vi "create_base_path.vi"(8 "folder name":string, 11 "folder":path) -> (3 "appended path":path)   [LabVIEW 2021]
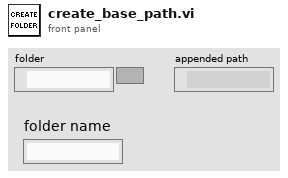
[diagram p1: front panel]
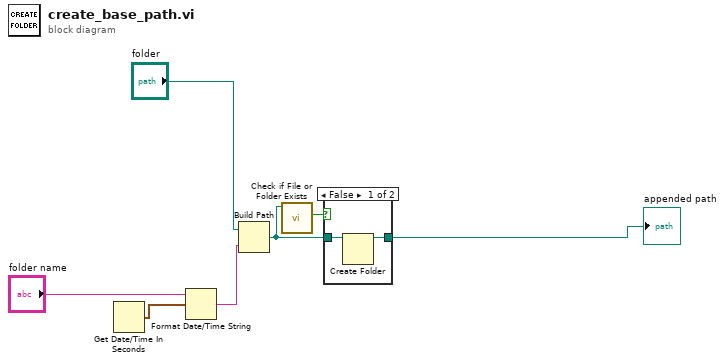
[diagram p0: block diagram]
diagram:
  n1 = Get Date/Time In Seconds() -> (seconds since 1Jan1904=w2:timestamp)
  n2 = Format Date/Time String(time format string (%c)="folder name", seconds (now)=w2) -> (date/time string=w1:string)  [unwired: 1 in]
  n3 = Build Path(base path="folder", name or relative path=w1) -> (appended path=w5:path)
  n4 = call <vilib>:"Check if File or Folder Exists.vi"("path"=w5) -> ("file or folder exists?"=w4:bool)  [unwired: 8 in, 2 out]
  n5 = case shown="False" w4 {
    tunnel: [w8 w10] -> w7
    tunnel: w5 -> [w9 w10]
    frame False {
      n6 = Create Folder(path (use dialog)=w9) -> (created path=w8:path)  [unwired: 2 in, 2 out]
    }
    frame True {
    }
  }
  "appended path" <- w7
